vi "Omniax_mDrive_Zonly_2017APXNoBK.vi"() -> ()   [LabVIEW 2015]
uses:
  <vilib>/Utility/file.llb/Read From Spreadsheet File (I64).vi
  <vilib>/Utility/file.llb/Read From Spreadsheet File (string).vi
  <userlib>/caLab/Private/Put_DBL_PV.vi
  <vilib>/Instr/_visa.llb/VISA Configure Serial Port (Instr).vi
  <userlib>/caLab/Private/Put_DBL-1D_PV-1D.vi
  <userlib>/caLab/Private/Get_PV-1D.vi
  <userlib>/caLab/Private/Put_I16-1D_PV-1D.vi
  <userlib>/caLab/Private/Put_I32_PV.vi
  <userlib>/caLab/Private/Get_PV.vi
  <userlib>/caLab/Private/Put_I32-1D_PV-1D.vi
  <vilib>/Utility/file.llb/Write To Spreadsheet File (I64).vi
panel:
  in  "APX:MZ_CHK local":bool
  out "APX:MZ_CHK":bool
  out "APX:MZ_STOP":bool
  out "retracted":bool
  out "facingup":bool
  out "gatevalve":bool
  in  "Remote":bool
  out "unsigned 8bit integer":u8
  out "SES is not busy":bool
  out "Status":bool
  in  "Pressure Overide":bool
  in  "Crash Override":bool
  in  "Is the gatevalve opened?":bool
  in  "Is the sample facinng up?":bool
  in  "Is the source retracted?":bool
  out "APX:MZ_MVG":bool
  out "inside HPC?":bool
  out "HPC01<0.001?":bool
  out "APX:V5 opened?":bool
  out "Isolated from GND?":bool
  out "APX:MZ_LIM":bool
  out "APX:MZ_RDY":bool
  in  "APX:MZ_RQ":dbl=10.0 min=290.0 max=355.7 step=0.1 format="%_6g"
  in  "APX:MZ_VLC_RQ":dbl=0.1 min=0.1 max=0.61 step=0.1
  out "Z Velocity SP step/sec":i32=102400 min=1 max=153600
  out "Z Step SP":i32=-20000 min=0 max=102400000 step=500
  out "Z Step PV":i32 max=2000
  out "Dev5 Voltage":dbl
  out "Z max step":i32
  in  "V5 position 15360000":i32
  out "APX:MZ_VLC_PV":dbl format="%.3f"
  out "Presets":i32[][](array[numeric])
  in  "stop":bool
  in  "Tab Control 3":enum32{"Console", "Reset", "Bypass"}(tab)
  out "APX:MZ status":string="Cancel"
  out "Status Message":string="HP cell pressure too high! or "
  in  "Reset Z Position mm":dbl
  out "Reset Z Motor Steps":i32
  in  "Reset":bool
  out "Z Position MV mm":dbl
  in  "Clear ZY":bool
  out "R Backlash steps/sec":i32
  out "R Backlash":i32
  out "R Holding Current %":i32
  out "R Run Current %":i32
  out "R offset deg":dbl
  out "R deg/rev":dbl
  out "R steps/rev":u32
  out "R velocity PV step/sec":i32
  out "Z COM PORT":refnum<visa-resource-name>="COM5"
  out "Z Backlash steps/sec":i32
  out "Z Backlash":i32
  out "Z Holding Current %":i32
  out "Z Run Current %":i32
  out "Z offset mm":dbl
  out "Z mm/rev":dbl
  out "Z steps/rev":u32
  out "Z  velocity PV step/sec":i32=102400
  out "Z MINPOS":i32=-94296
  out "Z MAXPOS":i32=-34296
  out "APX:MZ_PV":dbl format="%_5g"
  out "X velocity PV step/sec":i32
  out "X Backlash steps/sec":i32
  out "X Backlash":i32
  out "X Holding Current %":i32
  out "X Run Current %":i32
  out "X offset mm":dbl
  out "X mm/rev":dbl
  out "X steps/rev":u32
  out "Y Backlash steps/sec":i32
  out "Y Backlash":i32
  out "Y Holding Current %":i32
  out "Y Run Current %":i32
  out "Y offset mm":dbl
  out "Y mm/rev":dbl
  out "Y steps/rev":u32
  out "Y velocity PV step/sec":i32
  in  "STOP_button":bool
  # "APX:MZ"
  # "COM14"
  # "Prep to Main checkpoints"
  # "20 degree"
  # "290"
  # "60"
  # "355.7"
  # "10"
  # "289"
  # "55"
  # "102400000"
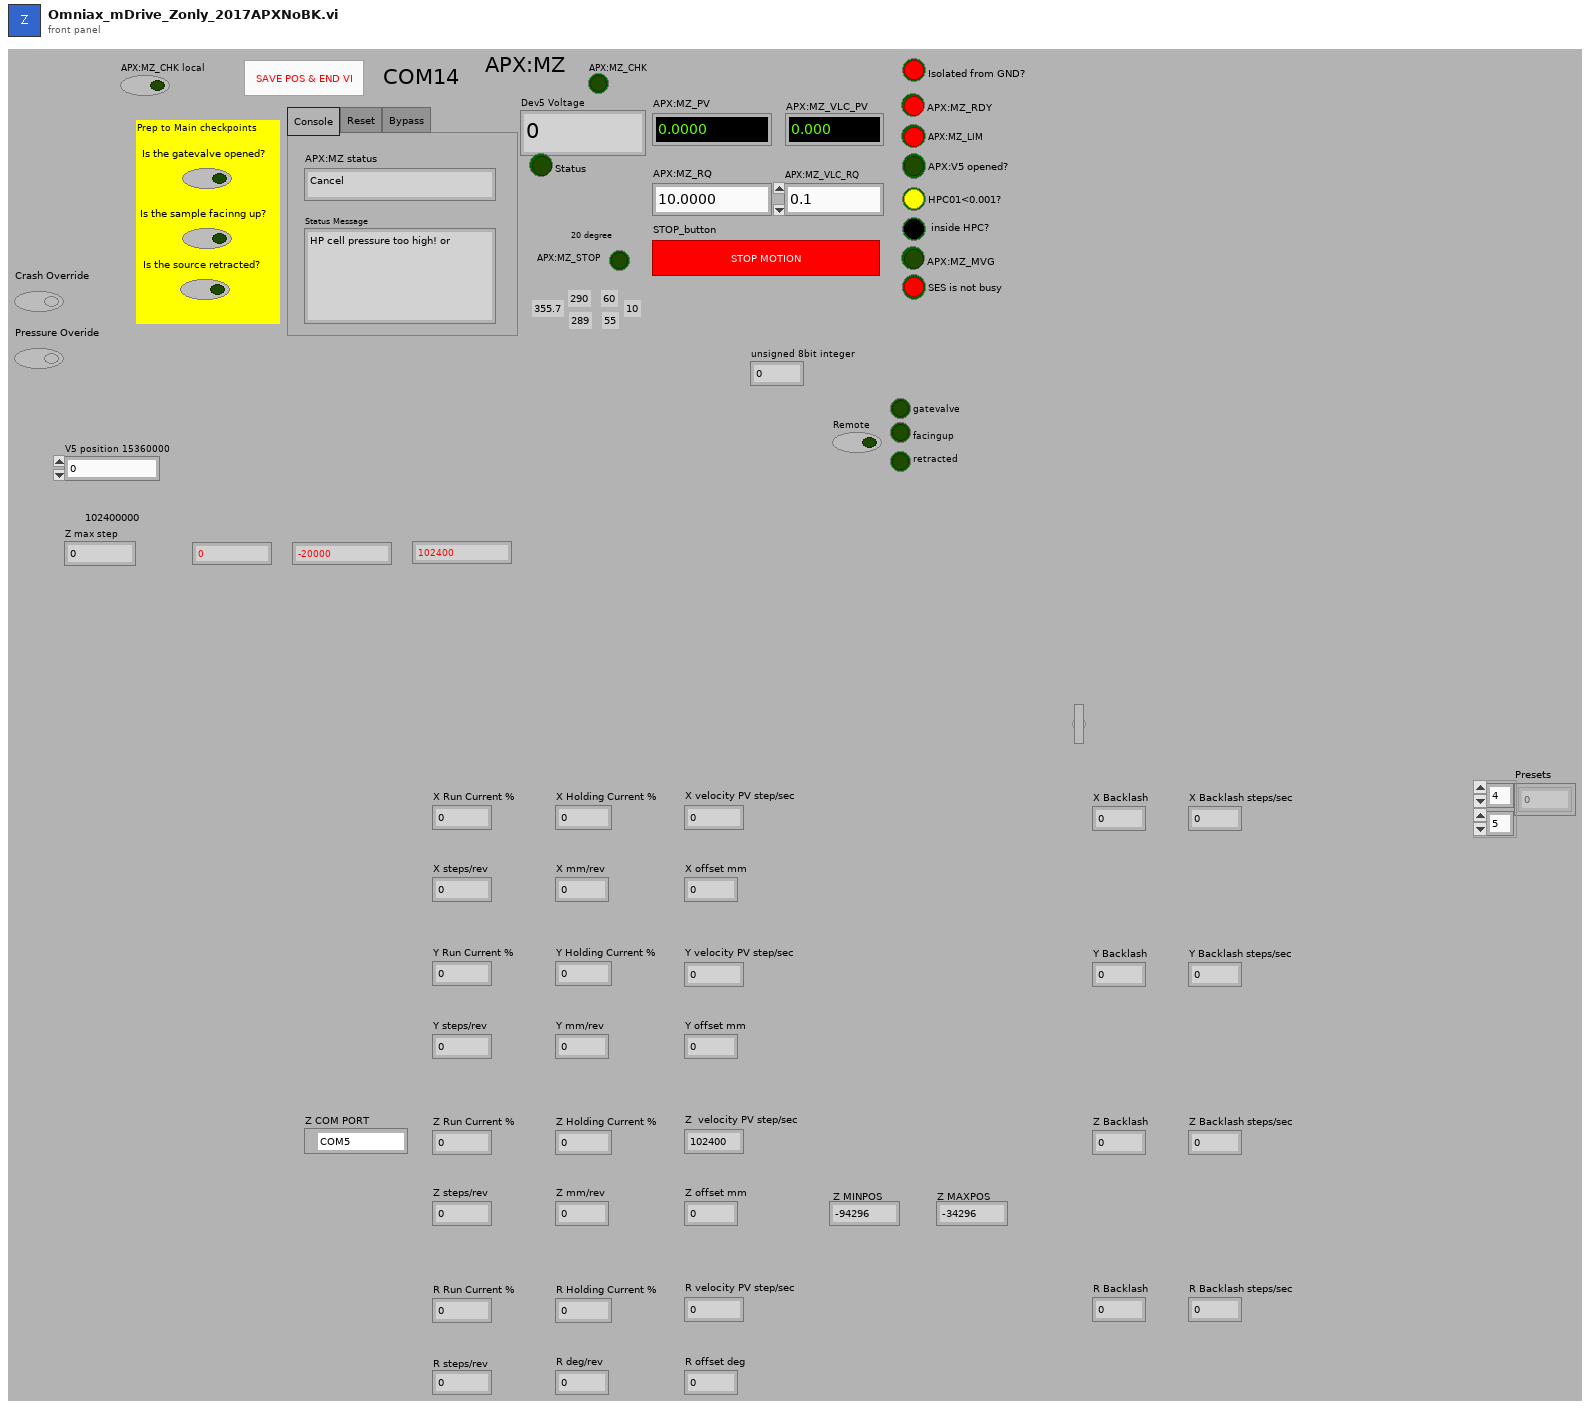
[diagram p1: front panel]
types:
  T1 = enum16{"Stop", "Reset", "Run Current", "Holding Current", "Accel Rate", "Decel Rate", "Move to Relative Position", "Move to Absolute Position", "Echo Mode", "Print Parameter", "Send String", "Microstep Resolution", "Set Current Position", "Max Velocity"}
  T2 = enum8{"Enabled", "Disabled", "Disabled and Grayed Out"}
  T3 = cluster{"first row[0]":i64, "first row[1]":i64, "first row[2]":i64, "first row[3]":i64, "first row[4]":i64, "first row[5]":i64, "first row[6]":i64, "first row[7]":i64, "first row[8]":i64}
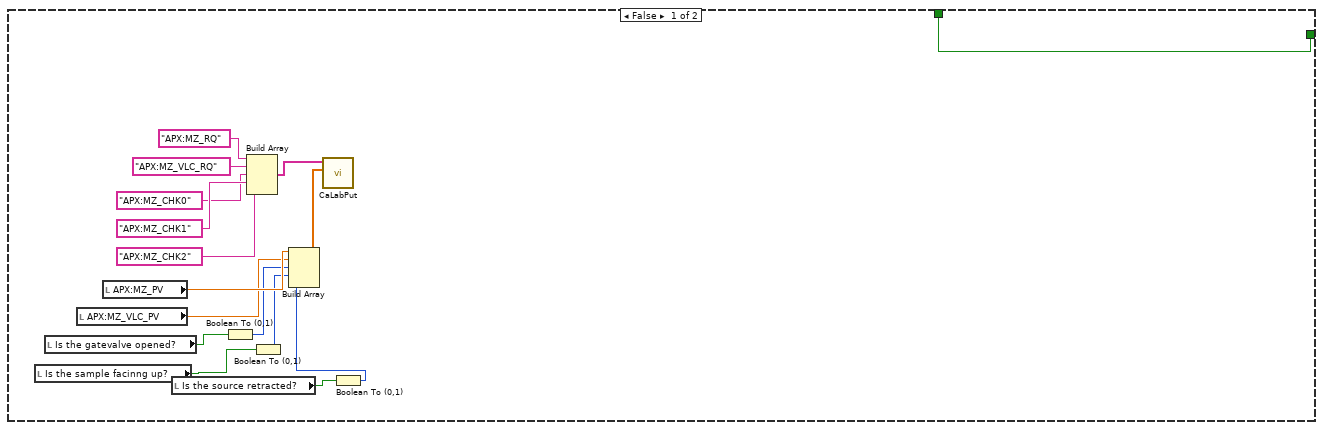
[diagram p3: hidden frame]
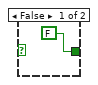
[diagram p7: hidden frame]
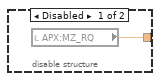
[diagram p8: hidden frame]
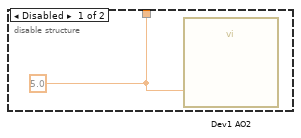
[diagram p9: hidden frame]
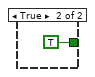
[diagram p10: hidden frame]
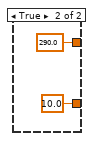
[diagram p11: hidden frame]
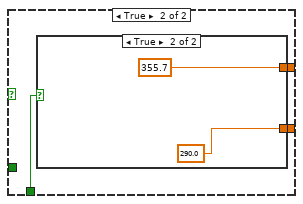
[diagram p12: hidden frame]
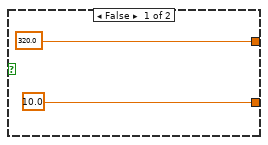
[diagram p13: hidden frame]
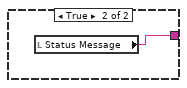
[diagram p16: hidden frame]
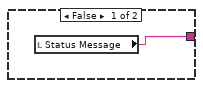
[diagram p17: hidden frame]
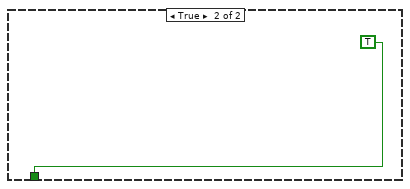
[diagram p18: hidden frame]
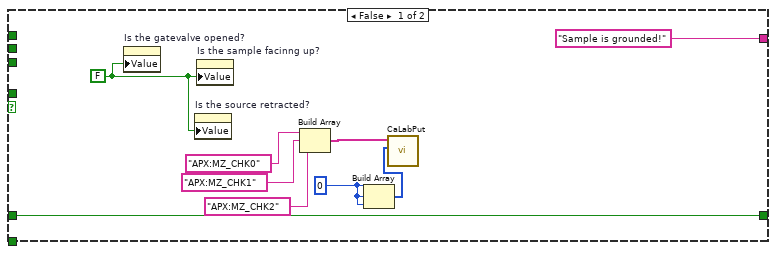
[diagram p19: hidden frame]
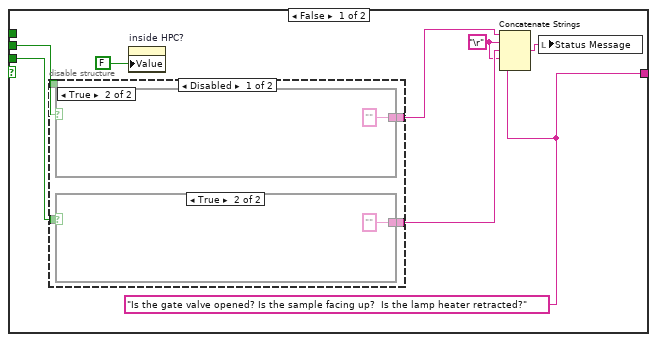
[diagram p20: hidden frame]
diagram:
  w4 = 0 ("dimension size")
  (unwired) 6144000 ("upper limit")
  (unwired) -6144000 ("lower limit")
  n1 = flat-sequence {
    tunnel: [w41] -> w23
    tunnel: [w42] -> w22
    tunnel: w23 -> [w57]
    tunnel: w22 -> [w56]
    tunnel: [w54] -> w2
    tunnel: [w52] -> w1
    tunnel: [w64] -> w27
    tunnel: [w60] -> w26
    tunnel: w2 -> [w61]
    tunnel: w1 -> [w60]
    tunnel: [w71] -> w38
    tunnel: [w73] -> w37
    tunnel: w27 -> [w72]
    tunnel: w26 -> [w74]
    tunnel: w38 -> [w81]
    tunnel: [w80] -> w36
    tunnel: w37 -> [w78]
    tunnel: [w79] -> w35
    tunnel: [w92] -> w34
    tunnel: [w93] -> w33
    tunnel: w36 -> [w91]
    tunnel: w35 -> [w90]
    tunnel: w34 -> [w103]
    tunnel: w33 -> [w102]
    tunnel: [w105] -> w32
    tunnel: [w104] -> w31
    tunnel: [w99] -> w30
    tunnel: [w112] -> w28
    tunnel: [w113] -> w29
    tunnel: w32 -> [w113]
    tunnel: w31 -> [w112]
    tunnel: w30 -> [w110]
    frame #0 {
      n2 = call-poly <userlib>:"CaLabPut.vi"("Value"=1.0, "PV Name"="SES:CalOff_RQ") -> ()  [unwired: 6 in, 4 out]
    }
    frame #1 {
      w49 = refnum<visa-resource-name> "COM14" ("COM PORT")
      w47 = u16 0 items=["None", "XON/XOFF", "RTS/CTS", "XON/XOFF & RTS/CTS", "DTR/DSR", "XON/XOFF & DTR/DSR"] ("flow control (0:none)")
      w46 = u16 10 items=["1.0"=10, "1.5"=15, "2.0"=20] ("stop bits (10: 1 bit)")
      # "Stop bits"
      n3 = call-poly "VISA Configure Serial Port"("VISA resource name"=w49, "timeout (10sec)"=u32 10000, "baud rate (9600)"=u32 9600, "data bits (8)"=u16 8, "parity (0:none)"=enum16{"None", "Odd", "Even", "Mark", "Space"}."None", "stop bits (10: 1 bit)"=w46, "flow control (0:none)"=w47) -> ("VISA resource name out"=w41:refnum<visa-resource-name>, "error out"=w42:errorcluster)  [unwired: 7 in]
      "Z COM PORT" <- w49
    }
    frame #2 {
      n4 = call "mDrive Send Command.vi"("error in (no error)"=w56, "Extra"="EM 2", "Command"=T1."Send String", "VISA resource name"=w57) -> ("error out"=w53:errorcluster, "VISA resource name out"=w55:refnum<visa-resource-name>)  [unwired: 3 in, 1 out]
      n5 = call "mDrive Send Command.vi"("error in (no error)"=w53, "Extra"="PR EE", "Command"=T1."Send String", "VISA resource name"=w55) -> ("error out"=w52:errorcluster, "VISA resource name out"=w54:refnum<visa-resource-name>)  [unwired: 3 in, 1 out]
    }
    frame #3 {
      n6 = Number To Decimal String(number=1000000) -> (decimal integer string=w62:string)  [unwired: 1 in]
      n7 = call "mDrive Send Command.vi"("Extra"=w62, "Command"=T1."Accel Rate", "VISA resource name"=w61) -> ("VISA resource name out"=w67:refnum<visa-resource-name>)  [unwired: 4 in, 2 out]
      n8 = call "mDrive Send Command.vi"("Extra"=w62, "Command"=T1."Decel Rate", "VISA resource name"=w67) -> ("VISA resource name out"=w64:refnum<visa-resource-name>)  [unwired: 4 in, 2 out]
    }
    frame #4 {
      # "Run Current %"
      n9 = property on="Z Run Current %" class="DigNum (strict)"() -> ("Value"=w69:i32)  [unwired: 2 in, 2 out]
      n10 = Number To Decimal String(number=w69) -> (decimal integer string=w70:string)  [unwired: 1 in]
      n11 = call "mDrive Send Command.vi"("error in (no error)"=w74, "Extra"=w70, "Command"=T1."Run Current", "VISA resource name"=w72) -> ("error out"=w73:errorcluster, "VISA resource name out"=w71:refnum<visa-resource-name>)  [unwired: 3 in, 1 out]
    }
    frame #5 {
      # "Holding Current %"
      n12 = property on="Z Run Current %" class="DigNum (strict)"() -> ("Value"=w76:i32)  [unwired: 2 in, 2 out]
      n13 = Number To Decimal String(number=w76) -> (decimal integer string=w77:string)  [unwired: 1 in]
      n14 = call "mDrive Send Command.vi"("error in (no error)"=w78, "Extra"=w77, "Command"=T1."Holding Current", "VISA resource name"=w81) -> ("error out"=w79:errorcluster, "VISA resource name out"=w80:refnum<visa-resource-name>)  [unwired: 3 in, 1 out]
    }
    frame #6 {
      # "Velocity Max"
      n15 = property on="Z Velocity SP step/sec" class="DigNum (strict)"() -> ("Value"=w89:i32)  [unwired: 2 in, 2 out]
      n16 = Number To Decimal String(number=w89) -> (decimal integer string=w88:string)  [unwired: 1 in]
      n17 = call "mDrive Send Command.vi"("error in (no error)"=w90, "Extra"=w88, "Command"=T1."Max Velocity", "VISA resource name"=w91) -> ("error out"=w86:errorcluster, "VISA resource name out"=w96:refnum<visa-resource-name>)  [unwired: 3 in, 1 out]
      n18 = call "mDrive Send Command.vi"("error in (no error)"=w86, "Extra"="VM", "Command"=T1."Print Parameter", "VISA resource name"=w96) -> ("error out"=w93:errorcluster, "read buffer"=w94:string, "VISA resource name out"=w92:refnum<visa-resource-name>)  [unwired: 3 in]
      n19 = Decimal String To Number(string=w94, offset=0) -> (number=w87:i32)  [unwired: 1 in, 1 out]
      n20 = local write "Remote"(FALSE ("Remote")) -> ()
      n21 = property on="Z  velocity PV step/sec" class="DigNum (strict)"("Val(Sgnl)"=w87) -> ()  [unwired: 2 in, 2 out]
    }
    frame #7 {
      # "PRINT POSITION"
      n22 = call "mDrive Send Command.vi"("error in (no error)"=w102, "Extra"="P", "Command"=T1."Print Parameter", "VISA resource name"=w103) -> ("error out"=w104:errorcluster, "read buffer"=w101:string, "VISA resource name out"=w105:refnum<visa-resource-name>)  [unwired: 3 in]
      n23 = Decimal String To Number(string=w101, offset=0) -> (number=w99:i32)  [unwired: 1 in, 1 out]
    }
    frame #8 {
      n24 = property on="Z Step SP" class="DigNum (strict)"("Val(Sgnl)"=w110) -> ()  [unwired: 2 in, 2 out]
      n25 = property on="Z Step SP" class="DigNum (strict)"() -> ("Maximum"=w107:dbl)  [unwired: 2 in, 2 out]
      n26 = property on="Z Step SP" class="DigNum (strict)"() -> ("Minimum"=w109:dbl)  [unwired: 2 in, 2 out]
      n27 = To Long Integer(number=w107) -> (32bit integer=w108:i32)
      "Z MAXPOS" <- w108
      n28 = To Long Integer(number=w109) -> (32bit integer=w106:i32)
      "Z MINPOS" <- w106
      n29 = In Range and Coerce(upper limit=w108, x=w110, lower limit=w106) -> (In Range?=w111:bool)  [unwired: 1 out]
      n30 = property on="APX:MZ_LIM" class="Bool (strict)"("Val(Sgnl)"=w111) -> ()  [unwired: 2 in, 2 out]
    }
  }
  n31 = flat-sequence {
    frame #0 {
      (unwired) 1.0 ("Data Entry Limits:Minimum")
      w117 = -3.0 ("R deg/rev")
      w115 = u32 51200 ("step/rev")
      n32 = To Double Precision Float(number=w115) -> (double precision float=w116:dbl)
      n33 = To Double Precision Float(number=10000 ("Value (Signaling)")) -> (double precision float=w121:dbl)
      n34 = Divide(x=w121, y=w116) -> (x/y=w120:dbl)
      n35 = Multiply(x=w120, y=w117) -> (x*y=w118:dbl)
      n36 = Absolute Value(x=w118) -> ()  [unwired: 1 out]
      "R offset deg" <- 0.0 ("R offset deg")
      "R deg/rev" <- w117
      "R steps/rev" <- w115
    }
  }
  n37 = flat-sequence {
    frame #0 {
      w125 = 0.2 ("Z mm/rev")
      w124 = u32 51200 ("step/rev")
      n38 = To Double Precision Float(number=153600 ("Value (Signaling)")) -> (double precision float=w129:dbl)
      n39 = To Double Precision Float(number=w124) -> (double precision float=w128:dbl)
      n40 = property on="Z Velocity SP step/sec" class="DigNum (strict)"("Val(Sgnl)"=51200 ("Value (Signaling)")) -> ()  [unwired: 2 in, 2 out]
      n41 = property on="Z Velocity SP step/sec" class="DigNum (strict)"("Minimum"=1.0 ("Data Entry Limits:Minimum")) -> ()  [unwired: 2 in, 2 out]
      n42 = Divide(x=w129, y=w128) -> (x/y=w127:dbl)
      n43 = property on="Z Velocity SP step/sec" class="DigNum (strict)"("Maximum"=w129) -> ()  [unwired: 2 in, 2 out]
      n44 = Multiply(x=w127, y=w125) -> ()  [unwired: 1 out]
      n45 = property on="APX:MZ_VLC_RQ" class="DigNum (strict)"("Val(Sgnl)"=0.2) -> ()  [unwired: 2 in, 2 out]
      "Z offset mm" <- 0.0 ("Z offset mm")
      "Z mm/rev" <- w125
      "Z steps/rev" <- w124
    }
  }
  n46 = disable-structure shown="Disabled" {
    frame Disabled {
      n47 = flat-sequence {
        frame #0 {
          w132 = FALSE ("Value (Signaling)")
          w135 = FALSE ("Value (Signaling)")
          w138 = FALSE ("Value (Signaling)")
          w139 = FALSE ("Value (Signaling)")
          "Z Backlash steps/sec" <- 25600 ("Z Backlash steps/sec")
          "Z Backlash" <- -51200 ("Z Backlash")
          "X Backlash steps/sec" <- 25600 ("Value (Signaling)")
          "X Backlash" <- 10240 ("Backlash2")
          "Y Backlash" <- -10240 ("Backlash2")
          "Y Backlash steps/sec" <- 25600 ("Value (Signaling)")
          "R Backlash steps/sec" <- 6400 ("R Backlash steps/sec")
          "R Backlash" <- -12800 ("R Backlash")
        }
      }
    }
    frame Enabled {
    }
  }
  n48 = flat-sequence {
    frame #0 {
      "Z Holding Current %" <- 20 ("Z Holding Current %")
      "Z Run Current %" <- 40 ("Z Run Current %")
      "X Run Current %" <- 40 ("Run Current %")
      "X Holding Current %" <- 20 ("Holding Current %")
      "Y Run Current %" <- 40 ("Run Current %")
      "Y Holding Current %" <- 20 ("Holding Current %")
      "R Holding Current %" <- 15 ("R Holding Current %")
      "R Run Current %" <- 80 ("R Run Current %")
    }
  }
  n49 = flat-sequence {
    frame #0 {
      (unwired) 0.1 ("Value (Signaling)")
      (unwired) FALSE ("Value (Signaling)")
      (unwired) T2."Disabled and Grayed Out" ("Disabled")
      (unwired) T2."Disabled and Grayed Out" ("Disabled")
      (unwired) 0.1 ("Value (Signaling)")
      (unwired) FALSE ("Value (Signaling)")
      (unwired) 0.1 ("Value (Signaling)")
      (unwired) FALSE ("Value (Signaling)")
      (unwired) 0.1 ("Value (Signaling)")
      (unwired) FALSE ("Value (Signaling)")
    }
  }
  n50 = flat-sequence {
    frame #0 {
      w154 = 0.2 ("MM/rev")
      w156 = u32 51200 ("step/rev")
      (unwired) 1.0 ("Data Entry Limits:Minimum")
      # "a=1000000"
      n51 = To Double Precision Float(number=128000 ("Value (Signaling)")) -> (double precision float=w157:dbl)
      n52 = To Double Precision Float(number=w156) -> (double precision float=w155:dbl)
      n53 = Divide(x=w157, y=w155) -> (x/y=w153:dbl)
      n54 = Multiply(x=w153, y=w154) -> ()  [unwired: 1 out]
      "X offset mm" <- 0.0 ("offset")
      "X steps/rev" <- w156
      "X mm/rev" <- w154
    }
  }
  n55 = flat-sequence {
    frame #0 {
      w161 = 0.2 ("MM/rev")
      w163 = u32 51200 ("step/rev")
      (unwired) 1.0 ("Data Entry Limits:Minimum")
      n56 = To Double Precision Float(number=128000 ("Value (Signaling)")) -> (double precision float=w164:dbl)
      n57 = To Double Precision Float(number=w163) -> (double precision float=w162:dbl)
      n58 = Divide(x=w164, y=w162) -> (x/y=w160:dbl)
      n59 = Multiply(x=w160, y=w161) -> ()  [unwired: 1 out]
      "Y offset mm" <- 0.0 ("offset")
      "Y steps/rev" <- w163
      "Y mm/rev" <- w161
    }
  }
  n60 = property on="Z Step SP" class="DigNum (strict)"("Minimum"=0 ("lower limit")) -> ()  [unwired: 2 in, 2 out]
  n61 = property on="V5 position 15360000" class="DigNum (strict)"("Value"=15360000 ("V5 position 15360000")) -> ()  [unwired: 2 in, 2 out]
  n62 = property on="Z Step SP" class="DigNum (strict)"("Maximum"=102400000 ("upper limit")) -> ()  [unwired: 2 in, 2 out]
  n63 = call-poly <vilib>:"Read From Spreadsheet File.vi"("file path (dialog if empty)"=path "T:/PAR/IMS/POSZ.TXT") -> ("first row"=w18:i64[])  [unwired: 6 in, 4 out]
  n64 = call-poly <vilib>:"Read From Spreadsheet File.vi"("file path (dialog if empty)"=path "T:/PAR/IMS/PRESET.TXT") -> ("all rows"=w10:string[][])  [unwired: 6 in, 4 out]
  n65 = Array To Cluster(array=w18) -> (cluster=w17:T3)
  n66 = Transpose 2D Array(2D array=w10) -> (transposed array=w11:string[][])
  n67 = Unbundle(w17) -> ("first row[2]"=w15:i64)  [unwired: 8 out]
  n68 = Delete From Array(array=w11, index (row)=0) -> (array with subset deleted=w13:string[][])  [unwired: 2 in, 1 out]
  n69 = property on="Reset Z Motor Steps" class="DigNum (strict)"("Val(Sgnl)"=w15) -> ()  [unwired: 2 in, 2 out]
  n70 = Transpose 2D Array(2D array=w13) -> (transposed array=w14:string[][])
  n71 = Decimal String To Number(string=w14) -> (number=w12:i32[][])  [unwired: 2 in, 1 out]
  n72 = Initialize Array(w4, w4, 4 ("dimension size")) -> (w7:i32[][])
  n73 = Build Array (concatenate)(w7, w12) -> (→"Presets":i32[][])
  n74 = while {
    tunnel: w29 -> [w181]
    tunnel: w28 -> [w180]
    tunnel: [w179] -> w21
    tunnel: [w178] -> w20
    tunnel: [w177] -> _
    tunnel: [w176] -> _
    i -> [w170]
    stop <- "stop" stop-if-true
    n75 = Quotient & Remainder(x=w170, y=2) -> (x-y*floor(x/y)=w173:i32)  [unwired: 1 out]
    n76 = Greater?(x=w170, y=2.0) -> ()  [unwired: 1 out]
    n77 = Equal To 0?(x=w173) -> (x = 0?=w174:bool)
    n78 = flat-sequence {
      frame #0 {
        n79 = local read "SES is not busy"() -> (w279:bool)
        n80 = disable-structure shown="Disabled" {
          frame Disabled {
            (unwired) 0
            n81 = local read "Is the gatevalve opened?"() -> (w285:bool)
            n82 = local read "Is the source retracted?"() -> (w287:bool)
            n83 = local read "Is the sample facinng up?"() -> (w286:bool)
            n84 = Build Array("APX:MZ_STOP", "APX:MZ_CHK") -> ()  [unwired: 1 in, 1 out]
            n85 = Build Array(w285, w286, w287) -> (w288:bool[])
            n86 = Boolean Array To Number(Boolean array=w288) -> ()  [unwired: 1 out]
          }
          frame Enabled {
          }
        }
        n87 = local read "inside HPC?"() -> (w280:bool)
        n88 = local read "Isolated from GND?"() -> (w281:bool)
        n89 = local read "APX:MZ_MVG"() -> (w282:bool)
        n90 = local read "APX:MZ_LIM"() -> (w275:bool)
        n91 = Build Array(w282, w281, w280, w279, w275) -> (w278:bool[])
        n92 = Boolean Array To Number(Boolean array=w278) -> (number=w277:u32)
        n93 = call-poly <userlib>:"CaLabPut.vi"("Value"=w277, "PV Name"="APX:MZ_STAT") -> ()  [unwired: 6 in, 4 out]
      }
    }
    n94 = case shown="True" w174 {
      tunnel: [FALSE ("Status") TRUE ("Status")] -> w168
      frame False {
      }
      frame True {
      }
    }
    "Status" <- w168
    n95 = case shown="True" "Remote" {
      tunnel: [w183 w199] -> w167
      tunnel: "APX:MZ_CHK local" -> [w183 _]
      frame False {
        n96 = local read "Is the sample facinng up?"() -> (w189:bool)
        n97 = local read "Is the gatevalve opened?"() -> (w190:bool)
        n98 = local read "APX:MZ_VLC_PV"() -> (w191:dbl)
        n99 = local read "APX:MZ_PV"() -> (w192:dbl)
        n100 = local read "Is the source retracted?"() -> (w188:bool)
        n101 = Boolean To (0,1)(Boolean=w190) -> (0, 1=w187:i16)
        n102 = Build Array("APX:MZ_RQ", "APX:MZ_VLC_RQ", "APX:MZ_CHK0", "APX:MZ_CHK1", "APX:MZ_CHK2") -> (w195:string[])
        n103 = Boolean To (0,1)(Boolean=w189) -> (0, 1=w186:i16)
        n104 = Boolean To (0,1)(Boolean=w188) -> (0, 1=w185:i16)
        n105 = Build Array(w192, w191, w187, w186, w185) -> (w184:dbl[])
        n106 = call-poly <userlib>:"CaLabPut.vi"("Values"=w184, "PV Names"=w195) -> ()  [unwired: 6 in, 4 out]
      }
      frame True {
        n107 = flat-sequence {
          tunnel: [w212] -> w203
          tunnel: w203 -> [w219]
          tunnel: [w224] -> w202
          tunnel: [w223] -> w201
          tunnel: [w222] -> w200
          tunnel: [w213] -> w199
          tunnel: w202 -> [w270]
          tunnel: w201 -> [w269]
          tunnel: w200 -> [w268]
          frame #0 {
            n108 = Build Array("APX:MZ_RQ", "APX:MZ_VLC_RQ", "APX:MZ_STOP", "APX:MZ_CHK0", "APX:MZ_CHK1", "APX:MZ_CHK2", "APX:MZ_CHK") -> (w211:string[])
            n109 = call-poly "CaLabGet.vi"("PV Names"=w211) -> ("Value Array (number)"=w212:dbl[][])  [unwired: 8 in, 6 out]
          }
          frame #1 {
            w221 = 0 ("index (col)")
            n110 = Index Array(array=w219, index (row)=0, index (col)=w221) -> (element=w254:dbl)
            n111 = Index Array(array=w219, index (row)=1, index (col)=w221) -> (element=w257:dbl)
            n112 = Index Array(array=w219, index (row)=2, index (col)=w221) -> (element=w248:dbl)
            n113 = Index Array(array=w219, index (row)=3, index (col)=w221) -> (element=w246:dbl)
            n114 = Index Array(array=w219, index (row)=4, index (col)=w221) -> (element=w237:dbl)
            n115 = Index Array(array=w219, index (row)=5, index (col)=w221) -> (element=w234:dbl)
            n116 = To Unsigned Byte Integer(number=w246) -> (unsigned 8bit integer=w245:u8)
            n117 = To Unsigned Byte Integer(number=w237) -> (unsigned 8bit integer=w238:u8)
            n118 = To Unsigned Byte Integer(number=w234) -> (unsigned 8bit integer=w235:u8)
            n119 = To Unsigned Byte Integer(number=w248) -> (unsigned 8bit integer=w232:u8)
            "unsigned 8bit integer" <- w232
            n120 = In Range and Coerce(upper limit=0.4, x=w257, lower limit=0.1) -> (coerced(x)=w250:dbl)  [unwired: 1 out]
            n121 = In Range and Coerce(upper limit=355.7, x=w254, lower limit=10.0) -> (coerced(x)=w251:dbl)  [unwired: 1 out]
            n122 = Number To Boolean Array(number=w245) -> (Boolean array=w241:bool[])
            n123 = Number To Boolean Array(number=w238) -> (Boolean array=w236:bool[])
            n124 = Number To Boolean Array(number=w235) -> (Boolean array=w233:bool[])
            n125 = local read "APX:MZ_VLC_RQ"() -> (w230:dbl)
            n126 = Index Array(array=w219, index (row)=6, index (col)=w221) -> (element=w218:dbl)
            n127 = Index Array(array=w241, index=0) -> (element=w224:bool)
            "gatevalve" <- w224
            n128 = Index Array(array=w236, index=0) -> (element=w223:bool)
            "facingup" <- w223
            n129 = Index Array(array=w233, index=0) -> (element=w222:bool)
            "retracted" <- w222
            n130 = To Unsigned Byte Integer(number=w218) -> (unsigned 8bit integer=w217:u8)
            n131 = Equal?(x=w217, y=u8 1) -> (x = y?=w213:bool)
            n132 = Number To Boolean Array(number=w232) -> (Boolean array=w227:bool[])
            n133 = local read "APX:MZ_RQ"() -> (w231:dbl)
            n134 = Index Array(array=w227, index=0) -> (element=→"APX:MZ_STOP":bool)
            n135 = local write "Is the source retracted?"(w222) -> ()
            n136 = local write "Is the gatevalve opened?"(w224) -> ()
            n137 = local write "Is the sample facinng up?"(w223) -> ()
            n138 = Equal?(x=w231, y=w251) -> (x = y?=w229:bool)
            n139 = And(x=w213, y=w229) -> (x .and. y?=w215:bool)
            n140 = Equal?(x=w230, y=w250) -> (x = y?=w228:bool)
            n141 = case shown="False" w215 {
              tunnel: w251 -> [w261 _]
              frame False {
                n142 = property on="APX:MZ_RQ" class="DigNum (strict)"("Val(Sgnl)"=w261) -> ()  [unwired: 2 in, 2 out]
              }
              frame True {
              }
            }
            n143 = And(x=w228, y=w213) -> (x .and. y?=w214:bool)
            n144 = case shown="False" w214 {
              tunnel: w250 -> [w260 _]
              frame False {
                n145 = property on="APX:MZ_VLC_RQ" class="DigNum (strict)"("Val(Sgnl)"=w260) -> ()  [unwired: 2 in, 2 out]
              }
              frame True {
              }
            }
          }
          frame #2 {
            n146 = Boolean To (0,1)(Boolean=w270) -> (0, 1=w267:i16)
            n147 = Boolean To (0,1)(Boolean=w269) -> (0, 1=w266:i16)
            n148 = Boolean To (0,1)(Boolean=w268) -> (0, 1=w265:i16)
            n149 = Build Array(i16 0 ("element"), w267, w266, w265) -> (w264:i16[])
            n150 = Build Array("APX:MZ_STOP", "APX:MZ_CHK0", "APX:MZ_CHK1", "APX:MZ_CHK2") -> (w271:string[])
            n151 = call-poly <userlib>:"CaLabPut.vi"("Values"=w264, "PV Names"=w271) -> ()  [unwired: 6 in, 4 out]
          }
        }
      }
    }
    "APX:MZ_CHK" <- w167
    n152 = event shown="[0] Timeout" {
      selector: _ -> [_ _ _ _ _ _]
      dyn-events: _ -> [_ _ _ _ _ _]
      timeout: 200 -> [_ _ _ _ _ _]
      tunnel: w181 -> [w317 _ _ w636 w711 w720]
      tunnel: w180 -> [w318 _ _ w635 w710 w719]
      tunnel: [w332 _ _ w633 w709 _] -> w179
      tunnel: [w331 _ _ w634 w708 _] -> w178
      tunnel: [_ _ _ _ _ w718] -> w177
      tunnel: [_ _ _ _ _ w717] -> w176
      event Timeout {
        n153 = event-data() -> ()  [unwired: 1 in, 2 out]
        n154 = property on="Is the gatevalve opened?" class="Bool (strict)"() -> ("Value"=w303:bool)  [unwired: 2 in, 2 out]
        n155 = property on="Is the sample facinng up?" class="Bool (strict)"() -> ("Value"=w304:bool)  [unwired: 2 in, 2 out]
        n156 = disable-structure shown="Enabled" {
          disable-tunnel: [w344 w345] -> _
          frame Disabled {
            n157 = local read "APX:MZ_RQ"() -> (w344:dbl)
          }
          frame Enabled {
            (unwired) "APX:MZ_RQ" ("PV Name")
            n158 = property on="APX:MZ_RQ" class="DigNum (strict)"() -> ("Value"=w345:dbl)  [unwired: 2 in, 2 out]
          }
        }
        n159 = property on="Is the sample facinng up?" class="Bool (strict)"() -> ("Value"=w312:bool)  [unwired: 2 in, 2 out]
        n160 = property on="Is the source retracted?" class="Bool (strict)"() -> ("Value"=w305:bool)  [unwired: 2 in, 2 out]
        n161 = property on="Isolated from GND?" class="Bool (strict)"() -> ("Value"=w322:bool)  [unwired: 2 in, 2 out]
        n162 = property on="Is the source retracted?" class="Bool (strict)"() -> ("Value"=w313:bool)  [unwired: 2 in, 2 out]
        n163 = And(x=w304, y=w305) -> (x .and. y?=w302:bool)
        n164 = And(x=w303, y=w302) -> (x .and. y?=w301:bool)
        n165 = local read "APX:MZ_VLC_PV"() -> (w295:dbl)
        n166 = case shown="True" w301 {
          tunnel: [w474 w475] -> w330
          frame False {
            n167 = property on="V5 position 15360000" class="DigNum (strict)"() -> ("Value"=w474:i32)  [unwired: 2 in, 2 out]
          }
          frame True {
            n168 = property on="Z Step SP" class="DigNum (strict)"() -> ("Maximum"=w475:dbl)  [unwired: 2 in, 2 out]
          }
        }
        "Z max step" <- w330
        n169 = Build Array("APX:MZ_PV" ("PV Name"), "APX:MZ_VLC_PV" ("PV Name")) -> (w292:string[])
        n170 = flat-sequence {
          tunnel: [w390] -> w314
          frame #0 {
            n171 = case shown="False" "Pressure Overide" {
              tunnel: [w392 TRUE] -> w390
              frame False {
                n172 = call-poly "CaLabGet.vi"("PV Name"="APX:HPC01") -> ("1rst Value (number)"=w407:dbl, "Error out"=w404:errorcluster)  [unwired: 8 in, 5 out]
                n173 = call-poly "CaLabGet.vi"("PV Name"="APX:V5_SOP", "Error in (no error)"=w404) -> ("1rst Value (number)"=w403:dbl, "Error out"=w396:errorcluster)  [unwired: 7 in, 5 out]
                n174 = call-poly "CaLabGet.vi"("PV Name"="SES:BUSY", "Error in (no error)"=w396) -> ("1rst Value (number)"=w395:dbl)  [unwired: 7 in, 6 out]
                n175 = Less?(x=w407, y=0.001) -> (x < y?=w401:bool)
                "HPC01<0.001?" <- w401
                n176 = Equal?(x=w395, y=0.0) -> (x = y?=w391:bool)
                "SES is not busy" <- w391
                n177 = Number To Boolean Array(number=w403) -> (Boolean array=w402:bool[])
                n178 = case shown="True" w401 {
                  tunnel: [w411 "HP cell pressure too high!"] -> w400
                  frame False {
                    n179 = local read "Status Message"() -> (w411:string)
                  }
                  frame True {
                  }
                }
                n180 = Index Array(array=w402) -> (element=w398:bool)  [unwired: 1 in]
                "APX:V5 opened?" <- w398
                n181 = case shown="False" w398 {
                  tunnel: ["HP Turbo GV is closed." w410] -> w399
                  frame False {
                  }
                  frame True {
                    n182 = local read "Status Message"() -> (w410:string)
                  }
                }
                n183 = Or(x=w401, y=w398) -> (x .or. y?=w393:bool)
                n184 = Or(x=w393, y=w391) -> (x .or. y?=w392:bool)
                n185 = local write "Status Message"(w400) -> ()
                n186 = local write "Status Message"(w399) -> ()
              }
              frame True {
              }
            }
          }
        }
        n187 = property on="Is the gatevalve opened?" class="Bool (strict)"() -> ("Value"=w319:bool)  [unwired: 2 in, 2 out]
        n188 = And(x=w312, y=w313) -> (x .and. y?=w311:bool)
        n189 = property on="APX:MZ_PV" class="DigNum (strict)"() -> ("Value"=w294:dbl)  [unwired: 2 in, 2 out]
        n190 = Build Array(w294, w295) -> (w293:dbl[])
        n191 = And(x=w319, y=w311) -> (x .and. y?=w325:bool)
        n192 = property on="inside HPC?" class="Bool (strict)"() -> ("Value"=w320:bool)  [unwired: 2 in, 2 out]
        n193 = flat-sequence {
          frame #0 {
            w349 = 10 ("number of samples")
            # "ai16 p0.16"
            # "Crash Sensing"
            n194 = call "Dev1 AI0"("number of samples"=w349) -> ("data"=w354:dynamicdata)  [unwired: 16 in, 2 out]
            n195 = disable-structure shown="Enabled" {
              disable-tunnel: [w361 5.0 ("data")] -> w360
              frame Disabled {
                w361 = 5.0 ("data")
                n196 = call "Dev1 AO2"("data"=w361) -> ()  [unwired: 17 in, 2 out]
              }
              frame Enabled {
                (unwired) bool[] [TRUE] ("data")
                n197 = local read "APX:MZ_CHK"() -> (w363:bool)
                n198 = Build Array(w363) -> (w362:bool[])
                n199 = call "Dev1 P1.7"("data"=w362) -> ()  [unwired: 17 in, 2 out]
              }
            }
            n200 = call "Convert from Dynamic Data"("Dynamic Data Type"=w354) -> ("Array"=w355:dbl[])  [unwired: 3 in]
            n201 = Add Array Elements(numeric array=w355) -> (sum=w353:dbl)
            n202 = Divide(x=w353, y=w349) -> (x/y=w352:dbl)
            n203 = Absolute Value(x=w352) -> (abs(x)=w356:dbl)
            "Dev5 Voltage" <- w356
            n204 = Multiply(x=w360, y=0.8) -> (x*y=w350:dbl)
            n205 = Greater?(x=w356, y=w350) -> (0:w357:bool)
            n206 = case shown="False" "Crash Override" {
              tunnel: [w365 TRUE] -> w358
              tunnel: w357 -> [w365 _]
              frame False {
              }
              frame True {
              }
            }
            n207 = local read "APX:MZ_STOP"() -> (w347:bool)
            n208 = Not(x=w347) -> (.not. x?=w346:bool)
            n209 = And(x=w346, y=w358) -> (x .and. y?=→"Isolated from GND?":bool)
          }
        }
        n210 = call-poly <userlib>:"CaLabPut.vi"("Values"=w293, "PV Names"=w292) -> ()  [unwired: 6 in, 4 out]
        n211 = Greater Or Equal?(x=w294, y=320.0) -> (x >= y?=w306:bool)
        n212 = And(x=w322, y=w325) -> (x .and. y?=w300:bool)
        n213 = Greater?(x=w294, y=55.0) -> (0:w326:bool)
        n214 = Greater?(x=w294, y=289.0) -> (0:w310:bool)
        n215 = case shown="True" w326 {
          tunnel: w322 -> [w422 _]
          tunnel: [w422 w428] -> w315
          tunnel: w300 -> [_ w428]
          tunnel: ["Sample is grounded!" w426] -> w323
          tunnel: w310 -> [_ w427]
          tunnel: w320 -> [_ w425]
          tunnel: w319 -> [_ w424]
          tunnel: w312 -> [_ w423]
          frame False {
            w415 = 0
            w420 = FALSE ("Open?")
            n216 = property on="Is the gatevalve opened?" class="Bool (strict)"("Value"=w420) -> ()  [unwired: 2 in, 2 out]
            n217 = property on="Is the source retracted?" class="Bool (strict)"("Value"=w420) -> ()  [unwired: 2 in, 2 out]
            n218 = property on="Is the sample facinng up?" class="Bool (strict)"("Value"=w420) -> ()  [unwired: 2 in, 2 out]
            n219 = Build Array("APX:MZ_CHK0" ("PV Name"), "APX:MZ_CHK1" ("PV Name"), "APX:MZ_CHK2" ("PV Name")) -> (w416:string[])
            n220 = Build Array(w415, w415, w415) -> (w414:i32[])
            n221 = call-poly <userlib>:"CaLabPut.vi"("Values"=w414, "PV Names"=w416) -> ()  [unwired: 6 in, 4 out]
          }
          frame True {
            n222 = case shown="True" w427 {
              tunnel: [w430 "Be careful, the sample enters into the HP cell!"] -> w426
              tunnel: w425 -> [_ w449]
              tunnel: w424 -> [w435 _]
              tunnel: w423 -> [w434 _]
              frame False {
                w431 = "\r"
                w430 = "Is the gate valve opened? Is the sample facing up?  Is the lamp heater retracted?"
                n223 = disable-structure shown="Disabled" {
                  disable-tunnel: w435 -> [w440 _]
                  disable-tunnel: w434 -> [w439 _]
                  disable-tunnel: [w438 _] -> w433
                  disable-tunnel: [w437 _] -> w432
                  frame Disabled {
                    n224 = case shown="True" w440 {
                      tunnel: ["Is the sample facing up?" ""] -> w438
                      frame False {
                      }
                      frame True {
                      }
                    }
                    n225 = case shown="True" w439 {
                      tunnel: ["Is the gate valve opened?" ""] -> w437
                      frame False {
                      }
                      frame True {
                      }
                    }
                  }
                  frame Enabled {
                  }
                }
                n226 = property on="inside HPC?" class="Bool (strict)"("Value"=FALSE ("inside HPC?")) -> ()  [unwired: 2 in, 2 out]
                n227 = Concatenate Strings(w433, w431, w432, w431, w430) -> (w429:string)
                n228 = local write "Status Message"(w429) -> ()
              }
              frame True {
                w445 = 0.1 ("APX:MZ_VLC_RQ")
                n229 = case shown="True" w449 {
                  frame False {
                  }
                  frame True {
                    n230 = local write "Status Message"("Sample is touching HPC!") -> ()
                  }
                }
                n231 = property on="APX:MZ_VLC_RQ" class="DigNum (strict)"("Value"=w445) -> ()  [unwired: 2 in, 2 out]
                n232 = property on="inside HPC?" class="Bool (strict)"("Value"=TRUE ("inside HPC?")) -> ()  [unwired: 2 in, 2 out]
                n233 = call-poly <userlib>:"CaLabPut.vi"("Value"=w445, "PV Name"="APX:MZ_VLC_RQ") -> ()  [unwired: 6 in, 4 out]
              }
            }
          }
        }
        n234 = case shown="False" w314 {
          tunnel: w318 -> [w383 w388]
          tunnel: [w382 w388] -> w316
          tunnel: w317 -> [w381 _]
          frame False {
            n235 = disable-structure shown="Disabled" {
              disable-tunnel: w383 -> [w386 _]
              disable-tunnel: [w385 _] -> w382
              disable-tunnel: w381 -> [w384 _]
              frame Disabled {
                n236 = call "mDrive Send Command.vi"("error in (no error)"=w386, "Command"=T1."Stop", "VISA resource name"=w384) -> ("error out"=w385:errorcluster)  [unwired: 4 in, 2 out]
              }
              frame Enabled {
              }
            }
          }
          frame True {
          }
        }
        n237 = Or(x=w314, y=w315) -> (x .or. y?=w299:bool)
        n238 = property on="Isolated from GND?" class="Bool (strict)"() -> ("Value"=w298:bool)  [unwired: 2 in, 2 out]
        n239 = And(x=w299, y=w298) -> (x .and. y?=w297:bool)
        n240 = case shown="False" w297 {
          tunnel: w317 -> [w458 w471]
          tunnel: [w457 w471] -> w329
          tunnel: [w455 w468] -> w328
          tunnel: w323 -> [w454 _]
          tunnel: w322 -> [w453 _]
          tunnel: [w452 w470] -> w321
          tunnel: w320 -> [_ w469]
          tunnel: w316 -> [w451 w468]
          frame False {
            n241 = case shown="True" w453 {
              tunnel: w454 -> [w459 w461]
              tunnel: [w459 "Be careful!"] -> w452
              frame False {
              }
              frame True {
                n242 = disable-structure shown="Disabled" {
                  disable-tunnel: [w464 _] -> w462
                  disable-tunnel: w461 -> [w463 _]
                  frame Disabled {
                    n243 = Two Button Dialog(message=w463, 1:"Cancel" ("F button name (\"Cancel\")"), 2:"OK" ("T button name (\"OK\")")) -> (T button?=w464:bool)
                  }
                  frame Enabled {
                  }
                }
                n244 = disable-structure shown="Disabled" {
                  disable-tunnel: w462 -> [w467 _]
                  frame Disabled {
                    n245 = property on="Is the gatevalve opened?" class="Bool (strict)"("Value"=w467) -> ()  [unwired: 2 in, 2 out]
                    n246 = property on="inside HPC?" class="Bool (strict)"("Value"=w467) -> ()  [unwired: 2 in, 2 out]
                    n247 = property on="Is the sample facinng up?" class="Bool (strict)"("Value"=w467) -> ()  [unwired: 2 in, 2 out]
                  }
                  frame Enabled {
                  }
                }
              }
            }
            n248 = call "mDrive Send Command.vi"("error in (no error)"=w451, "Command"=T1."Stop", "VISA resource name"=w458) -> ("error out"=w455:errorcluster, "VISA resource name out"=w457:refnum<visa-resource-name>)  [unwired: 4 in, 1 out]
          }
          frame True {
            n249 = case shown="False" w469 {
              tunnel: ["Normal" "In HPC! Be careful! "] -> w470
              frame False {
              }
              frame True {
              }
            }
          }
        }
        "APX:MZ status" <- w321
        n250 = case shown="False" w310 {
          tunnel: [w369 w376] -> w309
          tunnel: [w368 w375] -> w308
          tunnel: w306 -> [_ w374]
          tunnel: w300 -> [w367 _]
          frame False {
            n251 = case shown="False" w367 {
              tunnel: [60.0 ("Data Entry Limits:Maximum") 290.0 ("Data Entry Limits:Maximum")] -> w369
              tunnel: [10.0 ("Data Entry Limits:Minimum") 10.0 ("Data Entry Limits:Minimum")] -> w368
              frame False {
              }
              frame True {
              }
            }
          }
          frame True {
            n252 = case shown="True" w374 {
              tunnel: [320.0 ("Data Entry Limits:Maximum") 355.7 ("Data Entry Limits:Maximum")] -> w376
              tunnel: [10.0 ("Data Entry Limits:Minimum") 290.0 ("Data Entry Limits:Minimum")] -> w375
              frame False {
              }
              frame True {
              }
            }
          }
        }
        n253 = property on="APX:MZ_RQ" class="DigNum (strict)"("Maximum"=w309) -> ()  [unwired: 2 in, 2 out]
        n254 = property on="APX:MZ_RQ" class="DigNum (strict)"("Minimum"=w308) -> ()  [unwired: 2 in, 2 out]
        n255 = flat-sequence {
          tunnel: [w513] -> w343
          tunnel: [w492] -> w342
          tunnel: [w503] -> w341
          tunnel: [w483] -> w340
          tunnel: w329 -> [w482]
          tunnel: w328 -> [w481]
          tunnel: w343 -> [w517]
          tunnel: [w517] -> w339
          tunnel: w342 -> [w516]
          tunnel: [w516] -> w338
          tunnel: w341 -> [w515]
          tunnel: [w515] -> w337
          tunnel: w340 -> [w514]
          tunnel: [w514] -> w336
          tunnel: w339 -> [w520]
          tunnel: [w521] -> w335
          tunnel: w338 -> [w523]
          tunnel: [w522] -> w334
          tunnel: w337 -> [w519]
          tunnel: [w518] -> w333
          tunnel: w336 -> [w518]
          tunnel: w335 -> [w533]
          tunnel: w334 -> [w534]
          tunnel: w333 -> [w535]
          tunnel: [w532] -> w331
          tunnel: [w531] -> w332
          frame #0 {
            w487 = 0.1 ("Delay Time (s)")
            n256 = property on="Z Step SP" class="DigNum (strict)" props=["Maximum"]() -> ()  [unwired: 2 in, 3 out]
            n257 = call "mDrive Send Command.vi"("error in (no error)"=w481, "Extra"="P", "Command"=T1."Print Parameter", "VISA resource name"=w482) -> ("error out"=w508:errorcluster, "read buffer"=w512:string, "VISA resource name out"=w510:refnum<visa-resource-name>)  [unwired: 3 in]
            n258 = Decimal String To Number(string=w512, offset=0) -> (number=w494:i32)  [unwired: 1 in, 1 out]
            n259 = property on="Z Step SP" class="DigNum (strict)"() -> ("Minimum"=w506:dbl)  [unwired: 2 in, 2 out]
            n260 = property on="Z max step" class="DigNum (strict)"() -> ("Value"=w477:i32)  [unwired: 2 in, 2 out]
            n261 = To Long Integer(number=w494) -> (32bit integer=w495:i32)
            n262 = property on="Z Step PV" class="DigNum (strict)"("Val(Sgnl)"=w495) -> ()  [unwired: 2 in, 2 out]
            n263 = call "Time Delay17"("error in (no error)"=w508, "Delay Time (s)"=w487) -> ("error out"=w507:errorcluster)  [unwired: 9 in]
            n264 = To Long Integer(number=w506) -> (32bit integer=w505:i32)
            n265 = To Long Integer(number=w477) -> (32bit integer=w504:i32)
            n266 = property on="Z steps/rev" class="DigNum (strict)"() -> ("Value"=w501:u32)  [unwired: 2 in, 2 out]
            n267 = To Double Precision Float(number=w501) -> (double precision float=w502:dbl)
            n268 = In Range and Coerce(upper limit=w504, x=w495, lower limit=w505) -> (In Range?=w503:bool)  [unwired: 1 out]
            n269 = To Double Precision Float(number=w495) -> (double precision float=w496:dbl)
            n270 = Divide(x=w496, y=w502) -> (x/y=w500:dbl)
            n271 = property on="APX:MZ_LIM" class="Bool (strict)"("Val(Sgnl)"=w503) -> ()  [unwired: 2 in, 2 out]
            n272 = call "mDrive Send Command.vi"("error in (no error)"=w507, "Extra"="MV", "Command"=T1."Print Parameter", "VISA resource name"=w510) -> ("error out"=w509:errorcluster, "read buffer"=w478:string, "VISA resource name out"=w513:refnum<visa-resource-name>)  [unwired: 3 in]
            n273 = call "Time Delay16"("error in (no error)"=w509, "Delay Time (s)"=w487) -> ("error out"=w492:errorcluster)  [unwired: 9 in]
            n274 = Decimal String To Number(string=w478, offset=0 ("offset (0)")) -> (number=w486:i32)  [unwired: 1 in, 1 out]
            n275 = Not Equal?(x=w478, y="") -> (x != y?=w479:bool)
            n276 = property on="Z mm/rev" class="DigNum (strict)"() -> ("Value"=w499:dbl)  [unwired: 2 in, 2 out]
            n277 = property on="Z offset mm" class="DigNum (strict)"() -> ("Value"=w497:dbl)  [unwired: 2 in, 2 out]
            n278 = Multiply(x=w500, y=w499) -> (x*y=w498:dbl)
            n279 = Number To Boolean Array(number=w486) -> (Boolean array=w485:bool[])
            n280 = property on="APX:MZ_RDY" class="Bool (strict)"("Val(Sgnl)"=w479) -> ()  [unwired: 2 in, 2 out]
            n281 = Add(x=w498, y=w497) -> (x+y=w476:dbl)
            n282 = Index Array(array=w485, index=0) -> (element=w483:bool)
            n283 = property on="APX:MZ_PV" class="DigNum (strict)"("Val(Sgnl)"=w476) -> ()  [unwired: 2 in, 2 out]
            n284 = property on="APX:MZ_MVG" class="Bool (strict)"("Val(Sgnl)"=w483) -> ()  [unwired: 2 in, 2 out]
          }
          frame #1 {
          }
          frame #2 {
            n285 = case shown="False" w519 {
              tunnel: w520 -> [w526 w530]
              tunnel: [w527 w530] -> w521
              tunnel: [w528 w529] -> w522
              tunnel: w523 -> [w525 w529]
              frame False {
                n286 = call "mDrive Send Command.vi"("error in (no error)"=w525, "Command"=T1."Stop", "VISA resource name"=w526) -> ("error out"=w528:errorcluster, "VISA resource name out"=w527:refnum<visa-resource-name>)  [unwired: 4 in, 1 out]
              }
              frame True {
              }
            }
          }
          frame #3 {
            n287 = disable-structure shown="Enabled" {
              disable-tunnel: w535 -> [w541 _]
              disable-tunnel: w534 -> [w539 _]
              disable-tunnel: w533 -> [w538 _]
              disable-tunnel: [w537 _] -> w532
              disable-tunnel: [w536 _] -> w531
              frame Disabled {
                n288 = Implies(1:w541) -> (0:w540:bool, 2:w542:bool)
                n289 = case shown="False" w540 {
                  tunnel: w539 -> [w549 w602]
                  tunnel: w538 -> [w548 w603]
                  tunnel: [w547 w602] -> w537
                  tunnel: [w546 w603] -> w536
                  frame False {
                    # "Backlash"
                    n290 = flat-sequence {
                      tunnel: [w564] -> w561
                      tunnel: [w566] -> w560
                      tunnel: [w565] -> w559
                      tunnel: w549 -> [w563]
                      tunnel: w548 -> [w562]
                      tunnel: w561 -> [w574]
                      tunnel: [w574] -> w558
                      tunnel: w560 -> [w573]
                      tunnel: w559 -> [w572]
                      tunnel: [w571] -> w557
                      tunnel: [w570] -> w556
                      tunnel: [w569] -> w545
                      tunnel: w558 -> [w584]
                      tunnel: w557 -> [w583]
                      tunnel: w556 -> [w581]
                      tunnel: [w582] -> w555
                      tunnel: [w581] -> w554
                      tunnel: [w580] -> w551
                      tunnel: [w579] -> w550
                      tunnel: w545 -> [w579]
                      tunnel: w555 -> [w595]
                      tunnel: w554 -> [w588]
                      tunnel: [w595] -> w553
                      tunnel: [w594] -> w552
                      tunnel: w551 -> [w594]
                      tunnel: w550 -> [w590]
                      tunnel: [w589] -> w543
                      tunnel: w553 -> [w599]
                      tunnel: w552 -> [w598]
                      tunnel: [w597] -> w547
                      tunnel: [w596] -> w544
                      tunnel: w543 -> [w596]
                      tunnel: [w601] -> w546
                      tunnel: w544 -> [w601]
                      frame #0 {
                        n291 = property on="Z Backlash steps/sec" class="DigNum (strict)"() -> ("Value"=w564:i32)  [unwired: 2 in, 2 out]
                        n292 = Number To Decimal String(number=w564) -> (decimal integer string=w567:string)  [unwired: 1 in]
                        n293 = call "mDrive Send Command.vi"("error in (no error)"=w563, "Extra"=w567, "Command"=T1."Max Velocity", "VISA resource name"=w562) -> ("error out"=w565:errorcluster, "VISA resource name out"=w566:refnum<visa-resource-name>)  [unwired: 3 in, 1 out]
                      }
                      frame #1 {
                        n294 = property on="Z Backlash" class="DigNum (strict)"() -> ("Value"=w569:i32)  [unwired: 2 in, 2 out]
                        n295 = Number To Decimal String(number=w569) -> (decimal integer string=w575:string)  [unwired: 1 in]
                        n296 = call "mDrive Send Command.vi"("error in (no error)"=w572, "Extra"=w575, "Command"=T1."Move to Relative Position", "VISA resource name"=w573) -> ("error out"=w571:errorcluster, "VISA resource name out"=w570:refnum<visa-resource-name>)  [unwired: 3 in, 1 out]
                      }
                      frame #2 {
                        n297 = To Double Precision Float(number=w579) -> (double precision float=w577:dbl)
                        n298 = To Double Precision Float(number=w584) -> (double precision float=w586:dbl)
                        n299 = Absolute Value(x=w577) -> (abs(x)=w578:dbl)
                        n300 = Divide(x=w578, y=w586) -> (x/y=w587:dbl)
                        n301 = Add(x=w587, y=0.5) -> (x+y=w580:dbl)
                        n302 = call "Time Delay18"("error in (no error)"=w583, "Delay Time (s)"=w580) -> ("error out"=w582:errorcluster)  [unwired: 9 in]
                      }
                      frame #3 {
                        n303 = Negate(x=w590) -> (-x=w591:i32)
                        n304 = Number To Decimal String(number=w591) -> (decimal integer string=w592:string)  [unwired: 1 in]
                        n305 = call "mDrive Send Command.vi"("Extra"=w592, "Command"=T1."Move to Relative Position", "VISA resource name"=w588) -> ("VISA resource name out"=w589:refnum<visa-resource-name>)  [unwired: 4 in, 2 out]
                      }
                      frame #4 {
                        n306 = call "Time Delay19"("error in (no error)"=w599, "Delay Time (s)"=w598) -> ("error out"=w597:errorcluster)  [unwired: 9 in]
                      }
                      frame #5 {
                        w600 = FALSE ("Value (Signaling)")
                      }
                    }
                  }
                  frame True {
                  }
                }
              }
              frame Enabled {
              }
            }
          }
        }
      }
      event "Reset Z Position mm": Value Change {
        n307 = event-data() -> ()  [unwired: 1 in, 5 out]
        n308 = property on="Reset Z Position mm" class="DigNum (strict)"() -> ("Value"=w612:dbl)  [unwired: 2 in, 2 out]
        n309 = property on="Z offset mm" class="DigNum (strict)"() -> ("Value"=w604:dbl)  [unwired: 2 in, 2 out]
        n310 = Subtract(x=w612, y=w604) -> (x-y=w611:dbl)
        n311 = property on="Z steps/rev" class="DigNum (strict)"() -> ("Value"=w606:u32)  [unwired: 2 in, 2 out]
        n312 = property on="Z mm/rev" class="DigNum (strict)"() -> ("Value"=w605:dbl)  [unwired: 2 in, 2 out]
        n313 = Divide(x=w611, y=w605) -> (x/y=w610:dbl)
        n314 = To Double Precision Float(number=w606) -> (double precision float=w609:dbl)
        n315 = Multiply(x=w610, y=w609) -> (x*y=w608:dbl)
        n316 = To Long Integer(number=w608) -> (32bit integer=w607:i32)
        n317 = property on="Reset Z Motor Steps" class="DigNum (strict)"("Val(Sgnl)"=w607) -> ()  [unwired: 2 in, 2 out]
      }
      event "Z Velocity SP step/sec", "Z Step SP": Value Change {
        n318 = event-data() -> ()  [unwired: 1 in, 5 out]
        n319 = property on="Z Velocity SP step/sec" class="DigNum (strict)"() -> ("Value"=w624:i32)  [unwired: 2 in, 2 out]
        n320 = property on="Z steps/rev" class="DigNum (strict)"() -> ("Value"=w615:u32)  [unwired: 2 in, 2 out]
        n321 = property on="Z steps/rev" class="DigNum (strict)"() -> ("Value"=w622:u32)  [unwired: 2 in, 2 out]
        n322 = property on="Z Step SP" class="DigNum (strict)"() -> ("Value"=w617:i32)  [unwired: 2 in, 2 out]
        n323 = To Double Precision Float(number=w617) -> (double precision float=w618:dbl)
        n324 = To Double Precision Float(number=w615) -> (double precision float=w621:dbl)
        n325 = To Double Precision Float(number=w624) -> (double precision float=w625:dbl)
        n326 = To Double Precision Float(number=w622) -> (double precision float=w627:dbl)
        n327 = Divide(x=w618, y=w621) -> (x/y=w620:dbl)
        n328 = Divide(x=w625, y=w627) -> (x/y=w626:dbl)
        n329 = property on="Z mm/rev" class="DigNum (strict)"() -> ("Value"=w613:dbl)  [unwired: 2 in, 2 out]
        n330 = property on="Z offset mm" class="DigNum (strict)"() -> ("Value"=w614:dbl)  [unwired: 2 in, 2 out]
        n331 = Multiply(x=w620, y=w613) -> (x*y=w619:dbl)
        n332 = Multiply(x=w626, y=w613) -> (x*y=w623:dbl)
        n333 = property on="APX:MZ_VLC_PV" class="DigNum (strict)"("Val(Sgnl)"=w623) -> ()  [unwired: 2 in, 2 out]
        n334 = Add(x=w619, y=w614) -> (x+y=w616:dbl)
        n335 = property on="Z Position MV mm" class="DigNum (strict)"("Val(Sgnl)"=w616) -> ()  [unwired: 2 in, 2 out]
      }
      event "APX:MZ_RQ": Value Change {
        n336 = event-data() -> ()  [unwired: 1 in, 6 out]
        n337 = property on="APX:MZ_RQ" class="DigNum (strict)"() -> ("Value"=w632:dbl)  [unwired: 2 in, 2 out]
        n338 = property on="APX:MZ_PV" class="DigNum (strict)"() -> ("Value"=w631:dbl)  [unwired: 2 in, 2 out]
        n339 = Less?(x=w632, y=w631) -> (x < y?=w628:bool)
        n340 = property on="Isolated from GND?" class="Bool (strict)"() -> ("Value"=w630:bool)  [unwired: 2 in, 2 out]
        n341 = Or(x=w630, y=w628) -> (x .or. y?=w629:bool)
        n342 = case shown="True" w629 {
          tunnel: w636 -> [w638 w642]
          tunnel: w635 -> [w637 w641]
          tunnel: [w637 w640] -> w634
          tunnel: [w638 w639] -> w633
          frame False {
          }
          frame True {
            n343 = flat-sequence {
              tunnel: w641 -> [w651]
              tunnel: w642 -> [w652]
              tunnel: [w652] -> w650
              tunnel: [w651] -> w649
              tunnel: [w674] -> w648
              tunnel: [w673] -> w647
              tunnel: w650 -> [w676]
              tunnel: w649 -> [w675]
              tunnel: [w692] -> w646
              tunnel: [w691] -> w645
              tunnel: w648 -> [w690]
              tunnel: w647 -> [w689]
              tunnel: [w700] -> w644
              tunnel: [w699] -> w643
              tunnel: w646 -> [w698]
              tunnel: w645 -> [w697]
              tunnel: [w706] -> w640
              tunnel: [w707] -> w639
              tunnel: w644 -> [w707]
              tunnel: w643 -> [w705]
              frame #0 {
                (unwired) T2."Disabled and Grayed Out" ("Disabled")
                (unwired) T2."Disabled and Grayed Out" ("Disabled")
                n344 = flat-sequence {
                  frame #0 {
                    n345 = property on="APX:MZ_RQ" class="DigNum (strict)"() -> ("Value"=w664:dbl)  [unwired: 2 in, 2 out]
                    n346 = property on="Z offset mm" class="DigNum (strict)"() -> ("Value"=w665:dbl)  [unwired: 2 in, 2 out]
                    n347 = property on="APX:MZ_VLC_RQ" class="DigNum (strict)"() -> ("Value"=w658:dbl)  [unwired: 2 in, 2 out]
                    n348 = property on="Z steps/rev" class="DigNum (strict)"() -> ("Value"=w667:u32)  [unwired: 2 in, 2 out]
                    n349 = property on="Z mm/rev" class="DigNum (strict)"() -> ("Value"=w670:dbl)  [unwired: 2 in, 2 out]
                    n350 = Subtract(x=w664, y=w665) -> (x-y=w668:dbl)
                    n351 = property on="Z Velocity SP step/sec" class="DigNum (strict)"() -> ("Maximum"=w654:dbl)  [unwired: 2 in, 2 out]
                    n352 = property on="Z Velocity SP step/sec" class="DigNum (strict)"() -> ("Minimum"=w653:dbl)  [unwired: 2 in, 2 out]
                    n353 = Divide(x=w658, y=w670) -> (x/y=w659:dbl)
                    n354 = Divide(x=w668, y=w670) -> (x/y=w669:dbl)
                    n355 = To Double Precision Float(number=w667) -> (double precision float=w671:dbl)
                    n356 = property on="Z Step SP" class="DigNum (strict)"() -> ("Maximum"=w661:dbl)  [unwired: 2 in, 2 out]
                    n357 = property on="Z Step SP" class="DigNum (strict)"() -> ("Minimum"=w660:dbl)  [unwired: 2 in, 2 out]
                    n358 = Multiply(x=w659, y=w671) -> (x*y=w656:dbl)
                    n359 = Multiply(x=w669, y=w671) -> (x*y=w663:dbl)
                    n360 = In Range and Coerce(upper limit=w654, x=w656, lower limit=w653) -> (coerced(x)=w655:dbl)  [unwired: 1 out]
                    n361 = In Range and Coerce(upper limit=w661, x=w663, lower limit=w660) -> (coerced(x)=w662:dbl)  [unwired: 1 out]
                    n362 = To Long Integer(number=w655) -> (32bit integer=w657:i32)
                    n363 = To Long Integer(number=w662) -> (32bit integer=w666:i32)
                    n364 = property on="Z Velocity SP step/sec" class="DigNum (strict)"("Val(Sgnl)"=w657) -> ()  [unwired: 2 in, 2 out]
                    n365 = property on="Z Step SP" class="DigNum (strict)"("Val(Sgnl)"=w666) -> ()  [unwired: 2 in, 2 out]
                  }
                }
              }
              frame #1 {
                n366 = property on="Z Step SP" class="DigNum (strict)"() -> ("Value"=w684:i32)  [unwired: 2 in, 2 out]
                n367 = property on="Z Step PV" class="DigNum (strict)"() -> ("Value"=w683:i32)  [unwired: 2 in, 2 out]
                n368 = property on="Z Backlash" class="DigNum (strict)"() -> ("Value"=w672:i32)  [unwired: 2 in, 2 out]
                n369 = Subtract(x=w684, y=w683) -> (x-y=w682:i32)
                n370 = Sign(1:w682) -> (0:w681:i32)
                n371 = Sign(1:w672) -> (0:w680:i32)
                n372 = Multiply(x=w681, y=w680) -> (x*y=w679:i32)
                n373 = Equal?(x=w679, y=1) -> (x = y?=w677:bool)
                n374 = case shown="True" w677 {
                  tunnel: w676 -> [w686 w688]
                  tunnel: w675 -> [w685 w687]
                  tunnel: [w685 w687] -> w674
                  tunnel: [w686 w688] -> w673
                  frame False {
                    (unwired) FALSE ("Value (Signaling)")
                  }
                  frame True {
                    (unwired) TRUE ("Value (Signaling)")
                  }
                }
              }
              frame #2 {
                # "Velocity Setting"
                n375 = property on="Z Velocity SP step/sec" class="DigNum (strict)"() -> ("Value"=w693:i32)  [unwired: 2 in, 2 out]
                n376 = Number To Decimal String(number=w693) -> (decimal integer string=w694:string)  [unwired: 1 in]
                n377 = call "mDrive Send Command.vi"("error in (no error)"=w690, "Extra"=w694, "Command"=T1."Max Velocity", "VISA resource name"=w689) -> ("error out"=w691:errorcluster, "VISA resource name out"=w692:refnum<visa-resource-name>)  [unwired: 3 in, 1 out]
              }
              frame #3 {
                # "Move to Abs Position"
                n378 = call "Time Delay7"("error in (no error)"=w697) -> ("error out"=w696:errorcluster)  [unwired: 10 in]
                n379 = property on="Z Step SP" class="DigNum (strict)"() -> ("Value"=w703:i32)  [unwired: 2 in, 2 out]
                n380 = Number To Decimal String(number=w703) -> (decimal integer string=w702:string)  [unwired: 1 in]
                n381 = call "mDrive Send Command.vi"("error in (no error)"=w696, "Extra"=w702, "Command"=T1."Move to Absolute Position", "VISA resource name"=w698) -> ("error out"=w699:errorcluster, "VISA resource name out"=w700:refnum<visa-resource-name>)  [unwired: 3 in, 1 out]
              }
              frame #4 {
                n382 = call "Time Delay28"("error in (no error)"=w705, "Delay Time (s)"=0.1) -> ("error out"=w706:errorcluster)  [unwired: 9 in]
              }
            }
          }
        }
      }
      event "STOP_button": Mouse Down {
        n383 = event-data() -> ()  [unwired: 1 in, 7 out]
        n384 = flat-sequence {
          tunnel: [w715] -> w709
          tunnel: [w714] -> w708
          tunnel: w711 -> [w713]
          tunnel: w710 -> [w712]
          frame #0 {
            n385 = call "mDrive Send Command.vi"("error in (no error)"=w712, "Command"=T1."Stop", "VISA resource name"=w713) -> ("error out"=w714:errorcluster, "VISA resource name out"=w715:refnum<visa-resource-name>)  [unwired: 4 in, 1 out]
          }
        }
      }
      event "Reset": Mouse Down {
        n386 = event-data() -> ()  [unwired: 1 in, 7 out]
        n387 = flat-sequence {
          frame #0 {
          }
        }
        n388 = flat-sequence {
          frame #0 {
          }
        }
        n389 = flat-sequence {
          frame #0 {
          }
        }
        n390 = flat-sequence {
          tunnel: [w724] -> w718
          tunnel: [w723] -> w717
          tunnel: w720 -> [w722]
          tunnel: w719 -> [w721]
          frame #0 {
            n391 = property on="Reset Z Motor Steps" class="DigNum (strict)"() -> ("Value"=w725:i32)  [unwired: 2 in, 2 out]
            n392 = Number To Decimal String(number=w725) -> (decimal integer string=w726:string)  [unwired: 1 in]
            n393 = call "mDrive Send Command.vi"("error in (no error)"=w721, "Extra"=w726, "Command"=T1."Set Current Position", "VISA resource name"=w722) -> ("error out"=w723:errorcluster, "VISA resource name out"=w724:refnum<visa-resource-name>)  [unwired: 3 in, 1 out]
          }
        }
      }
    }
  }
  n394 = flat-sequence {
    tunnel: w21 -> [w734]
    tunnel: w20 -> [w732]
    tunnel: [w729] -> w19
    frame #0 {
      n395 = call "mDrive Send Command.vi"("error in (no error)"=w732, "Extra"="P", "Command"=T1."Print Parameter", "VISA resource name"=w734) -> ("error out"=w731:errorcluster, "read buffer"=w738:string, "VISA resource name out"=w733:refnum<visa-resource-name>)  [unwired: 3 in]
      n396 = call "Time Delay32"("error in (no error)"=w731) -> ("error out"=w728:errorcluster)  [unwired: 10 in]
      n397 = Decimal String To Number(string=w738, offset=0) -> (number=w730:i32)  [unwired: 1 in, 1 out]
      n398 = To Long Integer(number=w730) -> (32bit integer=w729:i32)
      n399 = call "mDrive Send Command.vi"("error in (no error)"=w728, "Command"=T1."Stop", "VISA resource name"=w733) -> ("error out"=w740:errorcluster, "VISA resource name out"=w741:refnum<visa-resource-name>)  [unwired: 4 in, 1 out]
      n400 = VISA Close(VISA resource name=w741, error in (no error)=w740) -> ()  [unwired: 1 out]
    }
  }
  n401 = flat-sequence {
    tunnel: w19 -> [w747]
    frame #0 {
      n402 = Build Array(0 ("element"), 0 ("element"), w747, 0 ("element")) -> (w745:i32[])
      n403 = call-poly <vilib>:"Write To Spreadsheet File.vi"("1D data"=w745, "file path (dialog if empty)"=path "T:/PAR/IMS/POSZ.TXT") -> ()  [unwired: 6 in, 1 out]
    }
    frame #1 {
    }
  }
